vi "Shift_005.vi"() -> ()   [LabVIEW 2019]
panel:
  in  "time threshold":dbl[unit]=5.0
  in  "Control Force":dbl[unit]=200.0
  in  "D":dbl[unit]=25.0
  out "Ep(tk)":dbl[unit][](array[numeric])
  out "Et(tk)":dbl[unit][](array[numeric])
  out "Ek(tk)":dbl[unit][](array[numeric])
  out "Et":cluster{dbl[unit][], dbl[unit][]}(graph)
  out "Ep":cluster{dbl[unit][], dbl[unit][]}(graph)
  out "Ek":cluster{dbl[unit][], dbl[unit][]}(graph)
  out "Et":dbl[unit][](graph)
  out "Ep":dbl[unit][](graph)
  out "Ek":dbl[unit][](graph)
  out "a":cluster{dbl[unit][], dbl[unit][]}(graph)
  out "v":cluster{dbl[unit][], dbl[unit][]}(graph)
  out "x":cluster{dbl[unit][], dbl[unit][]}(graph)
  out "time (tk)":dbl[unit][](array[numeric])
  out "a":dbl[unit][](graph)
  out "v":dbl[unit][](graph)
  out "x":dbl[unit][](graph)
  out "x(tk)":dbl[unit][](array[numeric])
  out "v(tk)":dbl[unit][](array[numeric])
  out "a(tk)":dbl[unit][](array[numeric])
  in  "M":dbl[unit]=100.0
  in  "k":dbl[unit]=1000.0
  in  "v0":dbl[unit]
  in  "x0":dbl[unit]=2.0
  in  "Dt":dbl[unit]=1e-05
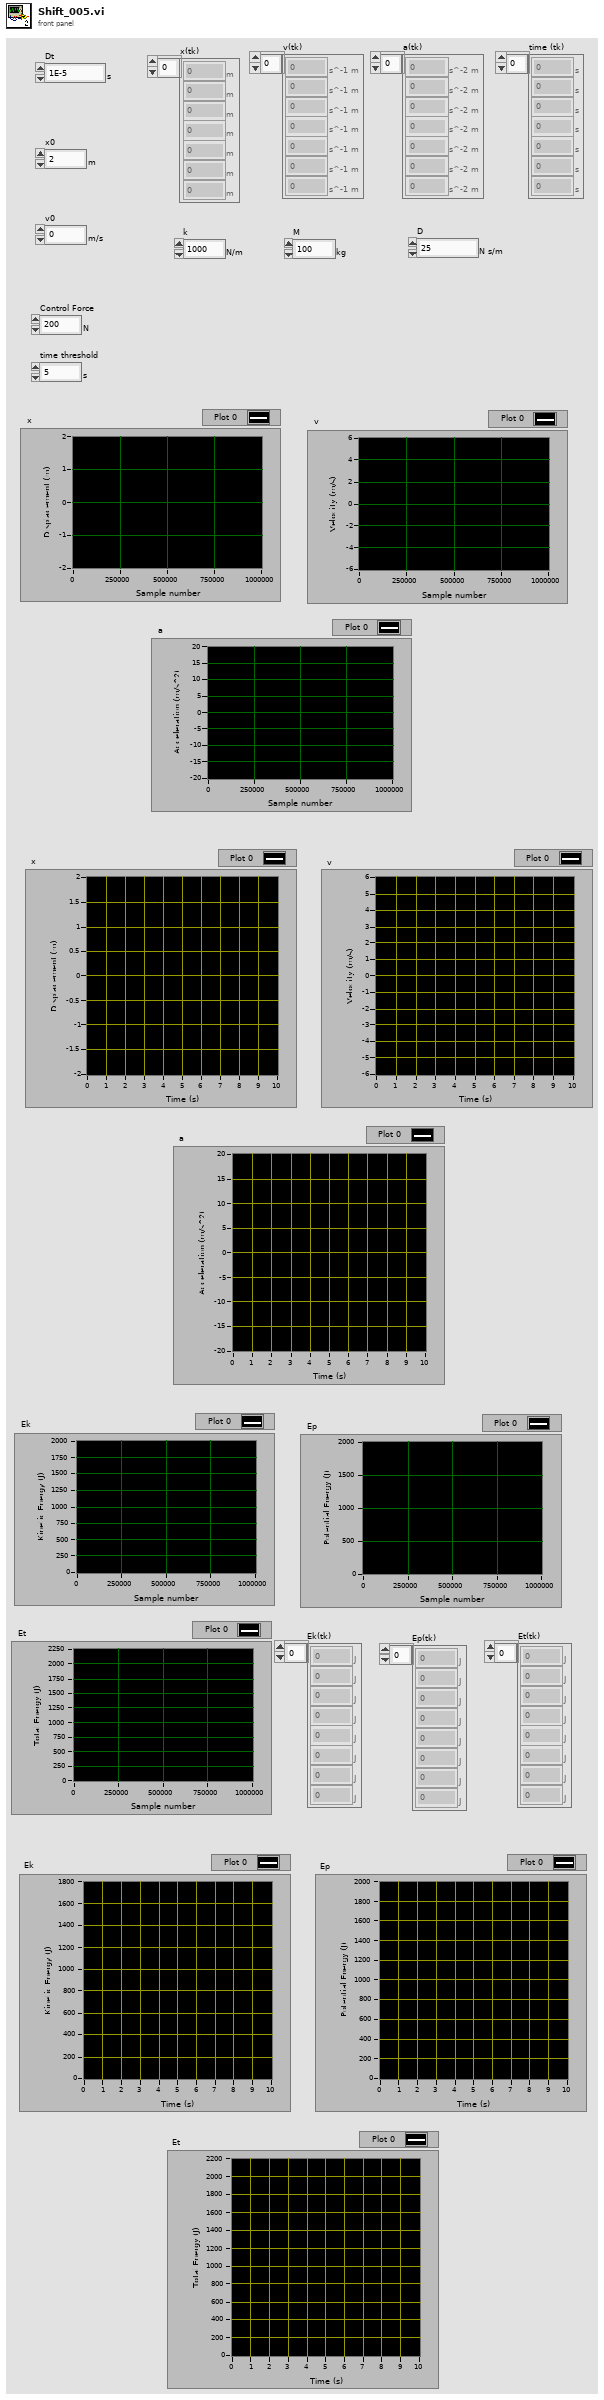
[diagram p1: front panel]
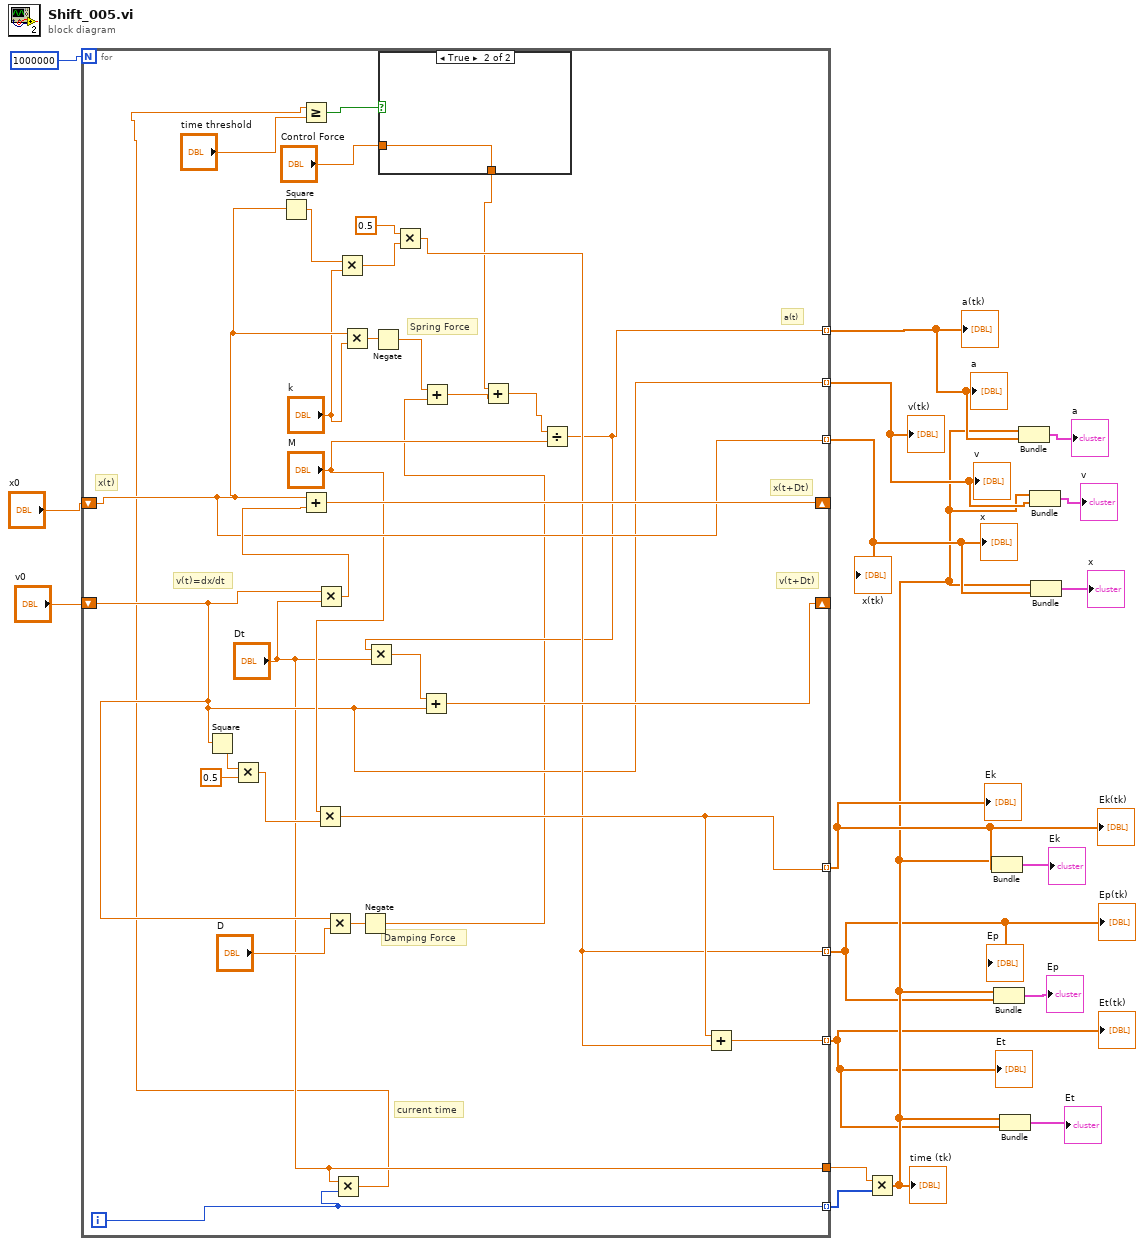
[diagram p0: block diagram]
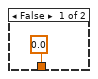
[diagram p2: hidden frame]
diagram:
  n1 = for {
    N: 1000000 -> [_]
    shift-right: [w49] -> _
    shift-left: "x0" -> [w43]
    shift-right: [w46] -> _
    shift-left: "v0" -> [w33]
    tunnel: [w29] -> w10 mode=indexing
    tunnel: [w33] -> w9 mode=indexing
    tunnel: [w43] -> w8 mode=indexing
    tunnel: [w24] -> w14 mode=indexing
    tunnel: ["Dt"] -> w15
    tunnel: [w38] -> w4 mode=indexing
    tunnel: [w35] -> w1 mode=indexing
    tunnel: [w37] -> w2 mode=indexing
    i -> [w24]
    # "current time"
    # "Spring Force"
    # "Damping Force"
    # "a(t)"
    # "v(t+Dt)"
    # "x(t+Dt)"
    # "v(t)=dx/dt"
    # "x(t)"
    n2 = Square(x=w33) -> (x^2=w44:dbl[unit])
    n3 = Multiply(x=w44, y=0.5) -> (x*y=w39:dbl[unit])
    n4 = Square(x=w43) -> (x^2=w42:dbl[unit])
    n5 = Multiply(x="M", y=w39) -> (x*y=w38:dbl[unit])
    n6 = Multiply(x=w33, y="Dt") -> (x*y=w50:dbl[unit])
    n7 = Add(x=w43, y=w50) -> (x+y=w49:dbl[unit])
    n8 = Multiply(x=w33, y="D") -> (x*y=w32:dbl[unit])
    n9 = Multiply(x="Dt", y=w24) -> (x*y=w20:dbl[unit])
    n10 = Greater Or Equal?(x=w20, y="time threshold") -> (x >= y?=w23:bool)
    n11 = Multiply(x=w42, y="k") -> (x*y=w41:dbl[unit])
    n12 = Multiply(x=w43, y="k") -> (x*y=w48:dbl[unit])
    n13 = Negate(x=w32) -> (-x=w28:dbl[unit])
    n14 = Negate(x=w48) -> (-x=w30:dbl[unit])
    n15 = case shown="True" w23 {
      tunnel: "Control Force" -> [_ w52]
      tunnel: [dbl[unit] 0.0 ("Control Force") w52] -> w21
      frame False {
      }
      frame True {
      }
    }
    n16 = Multiply(x=0.5, y=w41) -> (x*y=w35:dbl[unit])
    n17 = Add(x=w30, y=w28) -> (x+y=w27:dbl[unit])
    n18 = Add(x=w21, y=w27) -> (x+y=w26:dbl[unit])
    n19 = Divide(x=w26, y="M") -> (x/y=w29:dbl[unit])
    n20 = Multiply(x=w29, y="Dt") -> (x*y=w47:dbl[unit])
    n21 = Add(x=w47, y=w33) -> (x+y=w46:dbl[unit])
    n22 = Add(x=w38, y=w35) -> (x+y=w37:dbl[unit])
  }
  "a(tk)" <- w10
  "v(tk)" <- w9
  "x(tk)" <- w8
  "v" <- w9
  "a" <- w10
  "x" <- w8
  "Et" <- w2
  "Ek" <- w4
  "Ep" <- w1
  "Ek(tk)" <- w4
  "Et(tk)" <- w2
  "Ep(tk)" <- w1
  n23 = Multiply(x=w15, y=w14) -> (x*y=w3:dbl[unit][])
  "time (tk)" <- w3
  n24 = Bundle(w3, w4) -> (→"Ek":cluster{dbl[unit][], dbl[unit][]})  [unwired: 1 in]
  n25 = Bundle(w3, w1) -> (→"Ep":cluster{dbl[unit][], dbl[unit][]})  [unwired: 1 in]
  n26 = Bundle(w3, w2) -> (→"Et":cluster{dbl[unit][], dbl[unit][]})  [unwired: 1 in]
  n27 = Bundle(w3, w10) -> (→"a":cluster{dbl[unit][], dbl[unit][]})  [unwired: 1 in]
  n28 = Bundle(w3, w9) -> (→"v":cluster{dbl[unit][], dbl[unit][]})  [unwired: 1 in]
  n29 = Bundle(w3, w8) -> (→"x":cluster{dbl[unit][], dbl[unit][]})  [unwired: 1 in]
